vi "qMOD.vi"(0 "System no.":i32=1 min=1 max=4 step=1, 2 "ItemID to query":string[](array[string]), 3 "ModeID":i32[](array[numeric]), 4 "Without ItemIDs?":bool, 5 "error in":errorcluster) -> (14 "Value":i32[](array[numeric]), 16 "ItemID out":string[](array[string]), 17 "ModeID out":i32[](array[numeric]), 19 "error out":errorcluster)   [LabVIEW 2020]
doc: "Returns mode values for queried ItemIDs and ModeIDs. If Without ItemIDs? is TRUE, all available values for all Item/ModeIDs are returned. See driver manual for available ItemIDs and ModeIDs. \n\nE-870: For Without ItemIDs? = FALSE; only one ModeID for only one ItemID to query per command allowed."
uses:
  Communication/Global1.vi
panel:
  # "Returns mode values for queried ItemIDs and ModeIDs."
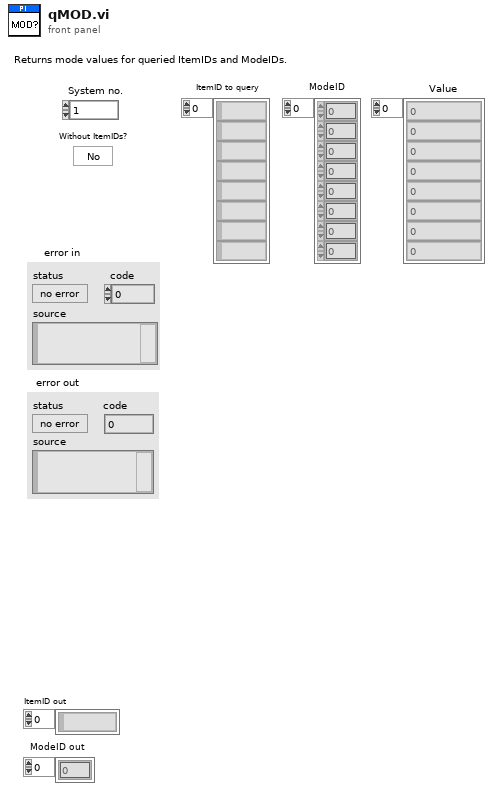
[diagram p1: front panel]
types:
  T1 = typedef "Syntax.ctl" = enum16{"GCS 1.0", "GCS 2.0", "GCS 3.0"}
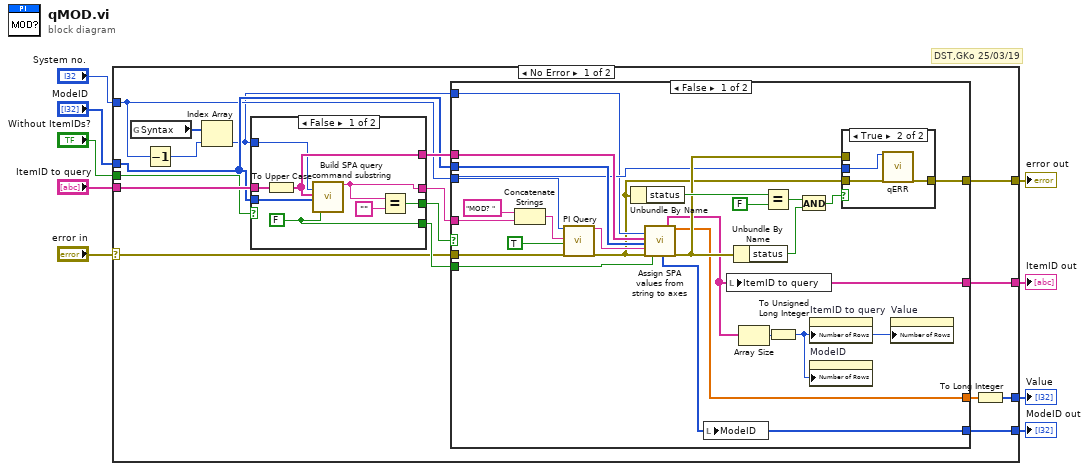
[diagram p0: block diagram]
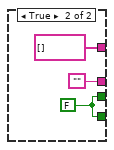
[diagram p2: hidden frame]
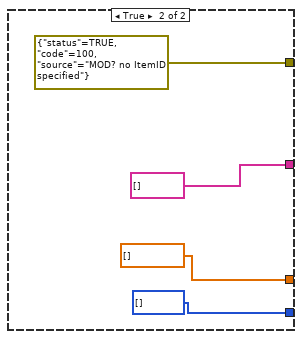
[diagram p4: hidden frame]
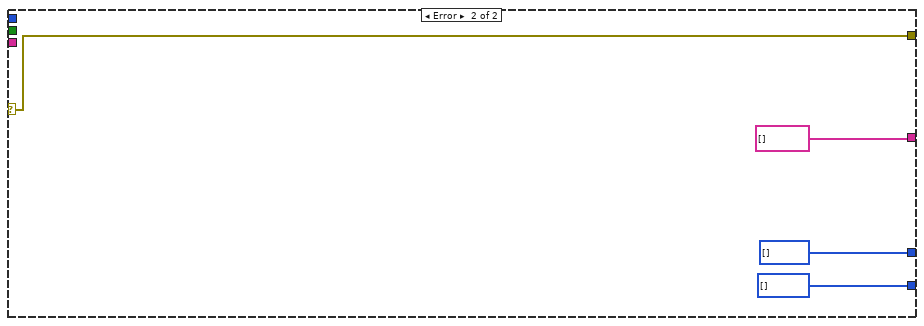
[diagram p5: hidden frame]
diagram:
  # "DST,GKo 25/03/19"
  n1 = case shown="No Error" "error in" {
    selector: "error in" -> [w11 w71]
    tunnel: "ItemID to query" -> [w26 _]
    tunnel: "System no." -> [w16 _]
    tunnel: "ModeID" -> [w23 _]
    tunnel: [w22 w71] -> w6
    tunnel: [w10 i32[] []] -> w5
    tunnel: "Without ItemIDs?" -> [w19 _]
    tunnel: [w14 string[] [] ("Queried axes out")] -> w3
    tunnel: [w13 i32[] [] ("Parameter no. out")] -> w2
    frame No Error {
      n2 = global read "Global1.vi" "Syntax"() -> (w17:T1[])
      n3 = Decrement(x=w16) -> (x-1=w18:i32)
      n4 = Index Array(array=w17, index=w18) -> (element=w15:T1)
      n5 = case shown="False" w19 {
        tunnel: w26 -> [w34 _]
        tunnel: [w33 "" ("Command substring")] -> w25
        tunnel: [w32 string[] [] ("Designator to query")] -> w24
        tunnel: w23 -> [w31 _]
        tunnel: [w30 w35] -> w21
        tunnel: w15 -> [w29 _]
        tunnel: [w27 w35] -> w12
        frame False {
          w27 = FALSE ("Parameter no. format \n(Decimal: FALSE)")
          n6 = To Upper Case(1:w34) -> (0:w32:string[])
          n7 = call "Build SPA query command substring.vi"("Syntax"=w29, "Axes to query"=w32, "Parameter number"=w31, "Parameter no. format \n(Decimal: FALSE)"=w27) -> ("Command substring"=w33:string)  [unwired: 3 in, 12 out]
          n8 = Equal?(x=w33, y="" ("x")) -> (x = y?=w30:bool)
        }
        frame True {
          w35 = FALSE
        }
      }
      n9 = case shown="False" w21 {
        tunnel: w11 -> [w48 _]
        tunnel: w25 -> [w58 _]
        tunnel: w24 -> [w57 _]
        tunnel: w16 -> [w47 _]
        tunnel: w23 -> [w56 _]
        tunnel: [w49 errorcluster {"status"=TRUE, "code"=100, "source"="MOD? no ItemID specified"} ("error out")] -> w22
        tunnel: [w41 dbl[] [] ("Parameter values")] -> w20
        tunnel: w15 -> [w46 _]
        tunnel: [w44 string[] [] ("Queried axes out")] -> w14
        tunnel: [w45 i32[] [] ("Parameter no. out")] -> w13
        tunnel: w12 -> [w42 _]
        frame False {
          n10 = Concatenate Strings("MOD? ", w58) -> (w59:string)
          n11 = call "PI Query.vi"("System no."=w47, "String to send"=w59, "Attach termination char.?"=TRUE ("Attach Linefeed?"), "error in"=w48) -> ("String read"=w39:string, "error out"=w38:errorcluster)  [unwired: 3 in, 11 out]
          n12 = Unbundle By Name(w38) -> ("status"=w55:bool)
          n13 = call "Assign SPA values from string to axes.vi"("Syntax"=w46, "Queried axes"=w57, "Parameter no."=w56, "Input string"=w39, "error in"=w38, "Parameter no. format \n(Decimal: FALSE)"=w42) -> ("Parameter no. out"=w45:i32[], "Queried axes out"=w44:string[], "Parameter values"=w41:dbl[], "error out"=w50:errorcluster)  [unwired: 2 in, 8 out]
          n14 = local write "ModeID"(w45) -> ()
          n15 = local write "ItemID to query"(w44) -> ()
          n16 = Unbundle By Name(w50) -> ("status"=w52:bool)
          n17 = Array Size(array=w44) -> (size(s)=w43:i32)
          n18 = Equal?(x=w55, y=FALSE) -> (x = y?=w53:bool)
          n19 = To Unsigned Long Integer(number=w43) -> (unsigned 32bit integer=w40:u32)
          n20 = And(x=w53, y=w52) -> (x .and. y?=w51:bool)
          n21 = property on="ItemID to query" class="Arr (strict)"("Number of Rows"=w40) -> ()  [unwired: 2 in, 2 out]
          n22 = property on="ModeID" class="Arr (strict)"("Number of Rows"=w40) -> ()  [unwired: 2 in, 2 out]
          n23 = case shown="True" w51 {
            tunnel: w50 -> [w62 _]
            tunnel: [w62 w64] -> w49
            tunnel: w47 -> [_ w65]
            tunnel: w38 -> [_ w63]
            frame False {
            }
            frame True {
              n24 = call "qERR.vi"("System no."=w65, "error in"=w63) -> ("error out"=w64:errorcluster)  [unwired: 17 out]
            }
          }
          n25 = property on="Value" class="Arr (strict)"("Number of Rows"=w40) -> ()  [unwired: 2 in, 2 out]
        }
        frame True {
        }
      }
      n26 = To Long Integer(number=w20) -> (32bit integer=w10:i32[])
    }
    frame Error {
    }
  }
  "error out" <- w6
  "Value" <- w5
  "ItemID out" <- w3
  "ModeID out" <- w2
